vi "Get Index Of First Unexplored Child.vi"(8 "Error In":errorcluster, 10 "DFS Node":T1, 11 "DFS Data":T3) -> (0 "Error Out":errorcluster, 2 "Index Of First Unexplored Child":i32, 3 "Was An Unexplored Child Found?":bool)   [LabVIEW 2022 SP3]
doc: "This VI returns the node index of the first unexplored child of an input node.\n\nIf the input node doesn't have children, or if all childred are fully explored, this VI returns -1."
uses:
  DFS Child Node (cluster).ctl
  DFS Node (cluster).ctl
  DFS Data (cluster).ctl
panel:
  # "Development\nControls or indicators that are useful for development or testing, but which are not outputs of the VI."
  # "Input\nInputs to the VI"
  # "Output\nOutputs of the VI"
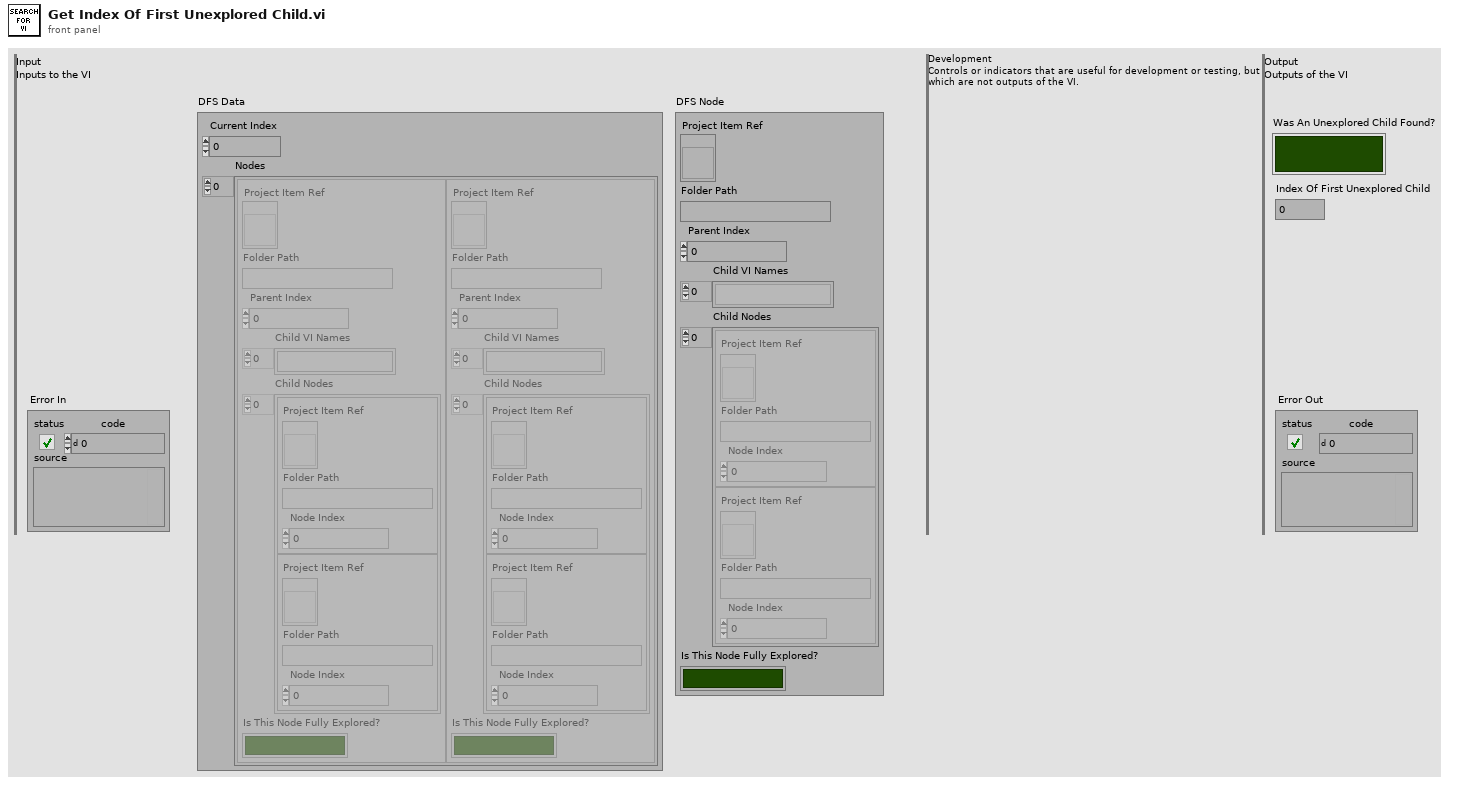
[diagram p1: front panel]
types:
  T1 = typedef "DFS Node (cluster).ctl" = cluster{"Project Item Ref":refnum<vi>, "Folder Path":string, "Parent Index":i32, "Child VI Names":string[], "Child Nodes":T2[], "Is This Node Fully Explored?":bool}
  T2 = typedef "DFS Child Node (cluster).ctl" = cluster{"Project Item Ref":refnum<vi>, "Folder Path":string, "Node Index":i32}
  T3 = typedef "DFS Data (cluster).ctl" = cluster{"Current Index":i32, "Nodes":T1[]}
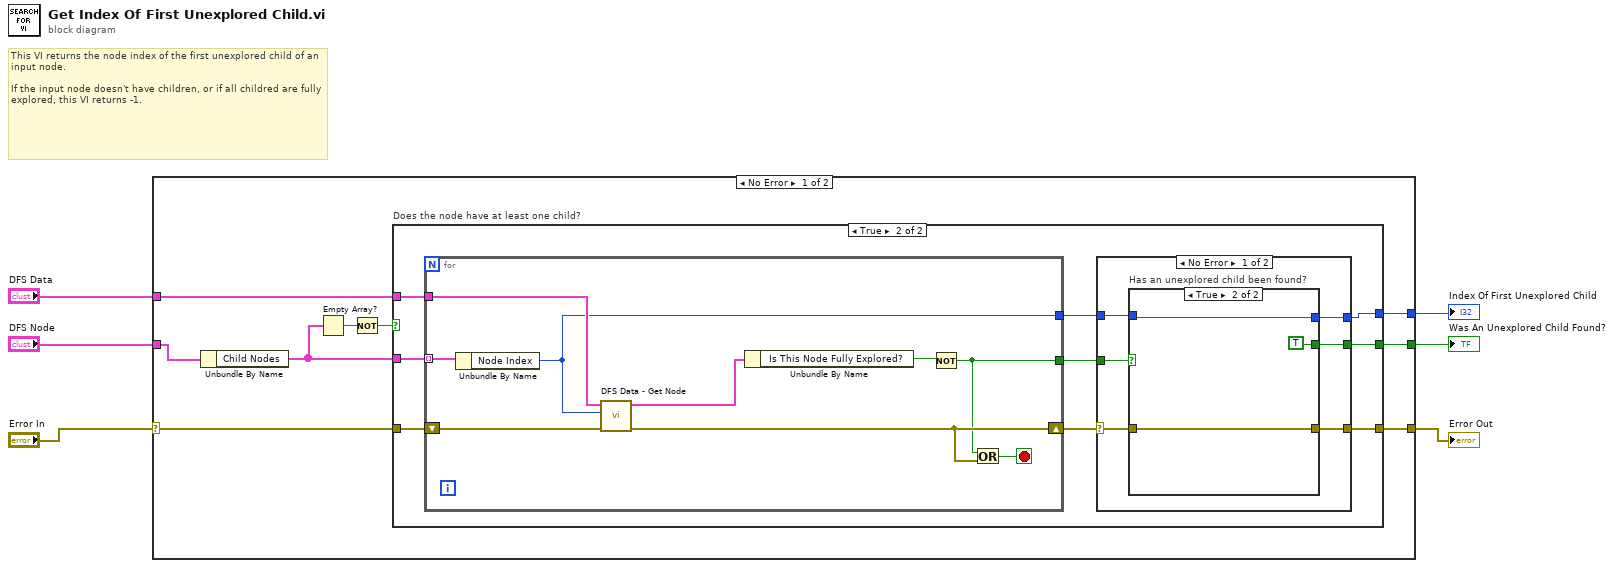
[diagram p0: block diagram]
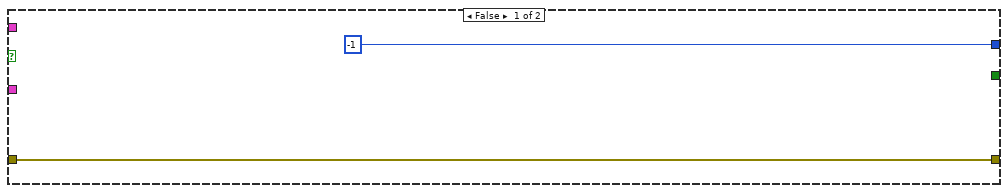
[diagram p2: hidden frame]
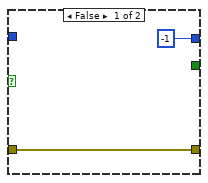
[diagram p3: hidden frame]
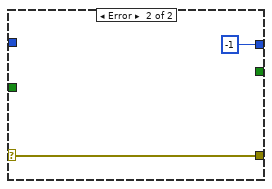
[diagram p4: hidden frame]
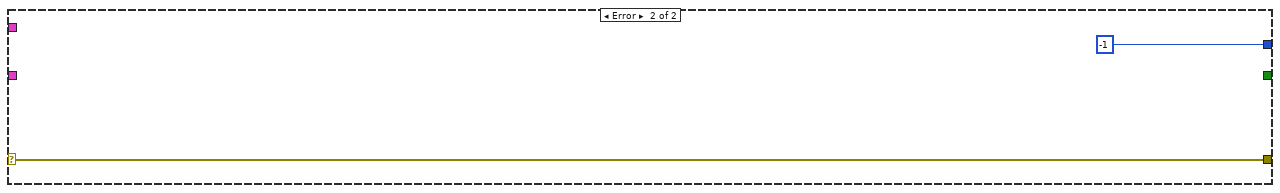
[diagram p5: hidden frame]
diagram:
  # "This VI returns the node index of the first unexplored child of an input node.\n\nIf the input node doesn't have children, or if all childred are fully explored, this VI returns -1."
  n1 = case shown="No Error" "Error In" {
    selector: "Error In" -> [w15 w50]
    tunnel: [w14 w50] -> w5
    tunnel: "DFS Data" -> [w12 _]
    tunnel: "DFS Node" -> [w13 _]
    tunnel: [w8 -1 ("Node Index")] -> w2
    tunnel: [w7 _] -> w1
    frame No Error {
      n2 = Unbundle By Name(w13) -> ("Child Nodes"=w11:T2[])
      n3 = Empty Array?(array=w11) -> (empty?=w10:bool)
      n4 = Not(x=w10) -> (.not. x?=w9:bool)
      n5 = case "Does the node have at least one child?" shown="True" w9 {
        tunnel: w15 -> [w17 w26]
        tunnel: [w17 w22] -> w14
        tunnel: w12 -> [_ w24]
        tunnel: w11 -> [_ w23]
        tunnel: [-1 w19] -> w8
        tunnel: [_ w18] -> w7
        frame False {
        }
        frame True {
          n6 = for {
            shift-right: [w43] -> w25
            shift-left: w26 -> [w46]
            tunnel: w23 -> [w48] mode=indexing
            tunnel: w24 -> [w47]
            tunnel: [w41] -> w20
            tunnel: [w40] -> w21
            stop <- w42 stop-if-true
            n7 = Unbundle By Name(w48) -> ("Node Index"=w41:i32)
            n8 = call "DFS Data - Get Node.vi"("Error In"=w46, "Node Index"=w41, "DFS Data"=w47) -> ("Error Out"=w43:errorcluster, "DFS Node"=w45:T1)  [unwired: 7 in]
            n9 = Unbundle By Name(w45) -> ("Is This Node Fully Explored?"=w44:bool)
            n10 = Not(x=w44) -> (.not. x?=w40:bool)
            n11 = Or(x=w40, y=w43) -> (x .or. y?=w42:bool)
          }
          n12 = case shown="No Error" w25 {
            selector: w25 -> [w32 w39]
            tunnel: [w31 w39] -> w22
            tunnel: w21 -> [w30 _]
            tunnel: w20 -> [w29 _]
            tunnel: [w28 -1 ("Node Index")] -> w19
            tunnel: [w27 _] -> w18
            frame No Error {
              n13 = case "Has an unexplored child been found?" shown="True" w30 {
                tunnel: w32 -> [w34 w37]
                tunnel: [w34 w37] -> w31
                tunnel: w29 -> [_ w36]
                tunnel: [-1 ("Node Index") w36] -> w28
                tunnel: [_ TRUE] -> w27
                frame False {
                }
                frame True {
                }
              }
            }
            frame Error {
            }
          }
        }
      }
    }
    frame Error {
    }
  }
  "Error Out" <- w5
  "Index Of First Unexplored Child" <- w2
  "Was An Unexplored Child Found?" <- w1
